vi "UIRef.vi"(8 "error in":errorcluster, 11 "channel in":refnum<class "Channel.lvclass">) -> (0 "error out":errorcluster, 2 "VI refnum":refnum<vi>, 3 "channel out":refnum<class "Channel.lvclass">)   [LabVIEW 2015, in "Channel.lvclass"]
uses:
  Channel.lvclass
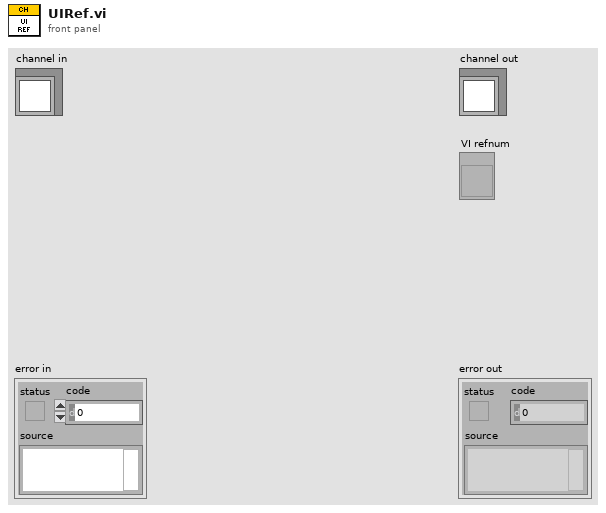
[diagram p1: front panel]
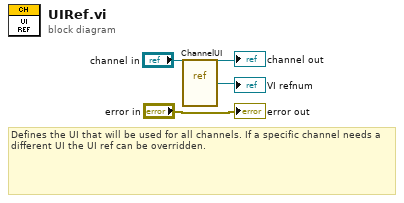
[diagram p0: block diagram]
diagram:
  # "Defines the UI that will be used for all channels. If a specific channel needs a different UI the UI ref can be overridden."
  n1 = vi-ref "ChannelUI.vi"() -> (→"VI refnum":refnum<vi>)
  "error out" <- "error in"
  "channel out" <- "channel in"
